vi "FTW-Regex.vi"(0 "Regular Expression":string, 5 "Input String":string, 9 "Starting Offset":i32, 11 "error in":errorcluster) -> (4 "Match":string, 6 "Submatches":string[](array[string]), 8 "Match Found?":bool, 10 "Offset after Match":i32, 15 "error out":errorcluster)   [LabVIEW 2013]
panel:
  out "Match Offsets":i32[](array[numeric])
  # "Inputs"
  # "Debug"
  # "Outputs"
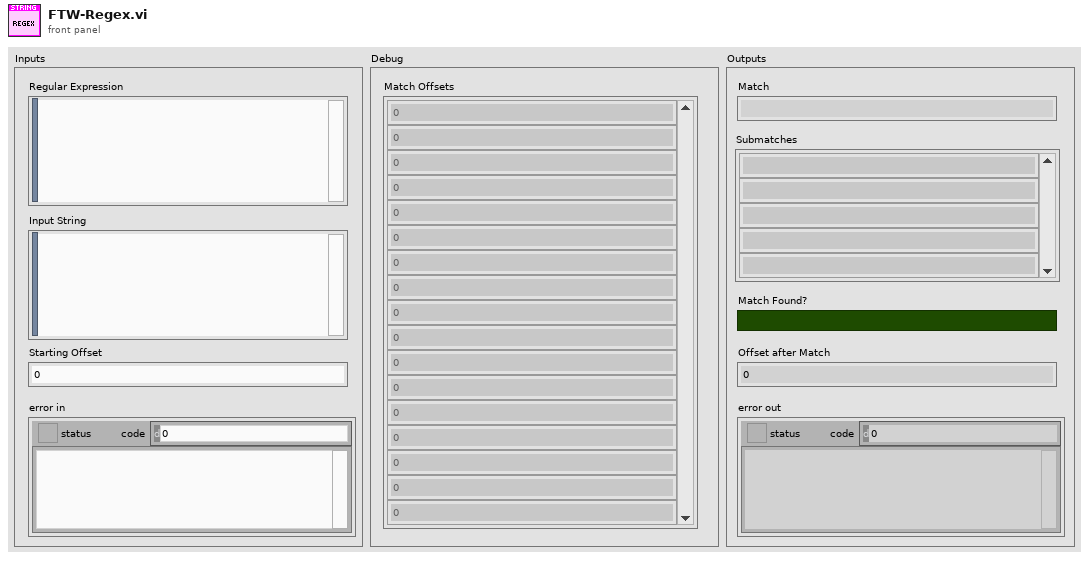
[diagram p1: front panel]
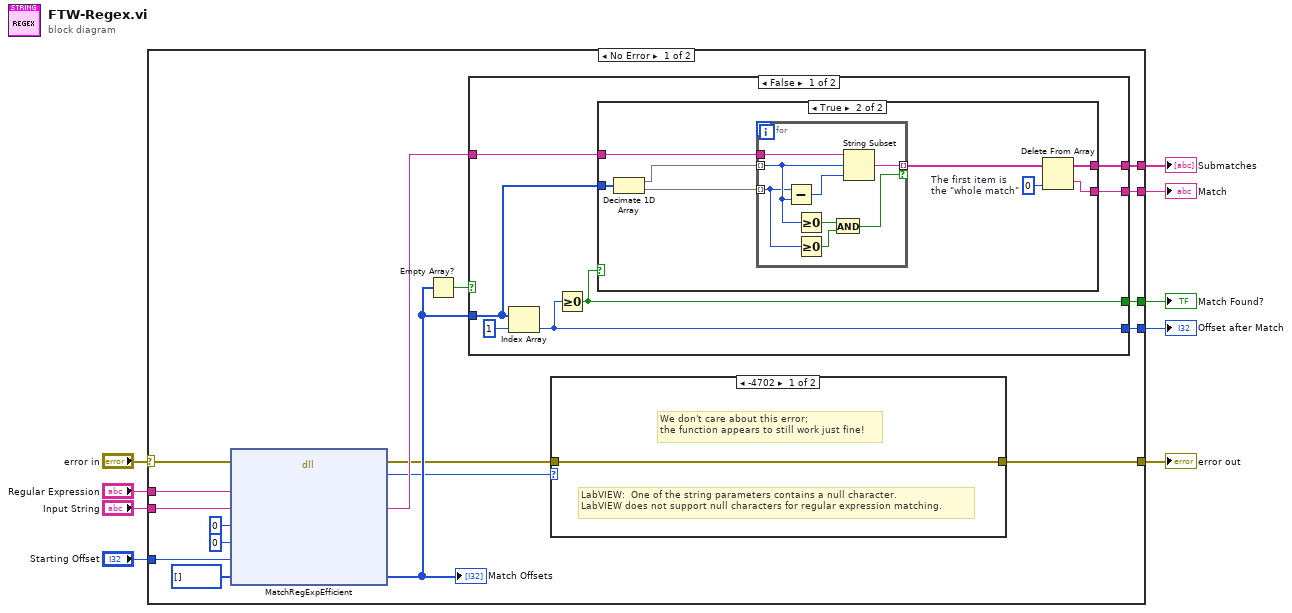
[diagram p0: block diagram]
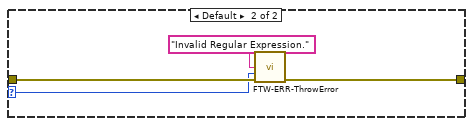
[diagram p2: hidden frame]
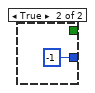
[diagram p4: hidden frame]
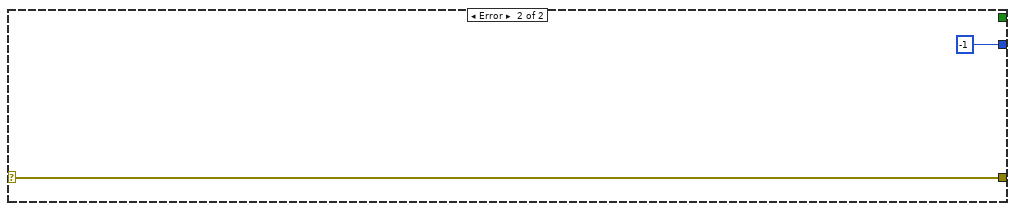
[diagram p5: hidden frame]
diagram:
  n1 = case shown="No Error" "error in" {
    selector: "error in" -> [w13 w56]
    tunnel: "Regular Expression" -> [w26 _]
    tunnel: [w25 _] -> w8
    tunnel: [w24 _] -> w7
    tunnel: [w11 w56] -> w6
    tunnel: "Starting Offset" -> [w23 _]
    tunnel: [w22 -1] -> w4
    tunnel: [w21 _] -> w3
    tunnel: "Input String" -> [w20 _]
    frame No Error {
      n2 = dll-call lib="LabVIEW" fn="MatchRegExpEfficient"(error in=w13, "Regular Expression"=w26, "Subject"=w20, "Ignore Case?"=0, "Multiline?"=0, "Starting Offset"=w23, "Match Offsets"=i32[] []) -> (error out=w12:errorcluster, "Return"=w10:i32, "Subject"=w19:string, "Match Offsets"=w15:i32[])  [unwired: 6 in, 1 out]
      "Match Offsets" <- w15
      n3 = Empty Array?(array=w15) -> (empty?=w14:bool)
      n4 = case shown="False" w14 {
        tunnel: [w38 _] -> w25
        tunnel: [w37 _] -> w24
        tunnel: [w35 -1] -> w22
        tunnel: [w34 _] -> w21
        tunnel: w19 -> [w33 _]
        tunnel: w15 -> [w32 _]
        frame False {
          n5 = Index Array(array=w32, index=1) -> (element=w35:i32)
          n6 = Greater Or Equal To 0?(x=w35) -> (x >= 0?=w34:bool)
          n7 = case shown="True" w34 {
            tunnel: w33 -> [_ w46]
            tunnel: [_ w42] -> w38
            tunnel: [_ w41] -> w37
            tunnel: w32 -> [_ w39]
            frame False {
            }
            frame True {
              w43 = 0  # The first item is the "whole match"
              n8 = Decimate 1D Array(w39) -> (w45:i32[], w40:i32[])
              n9 = for {
                tunnel: w46 -> [w54]
                tunnel: [w53] -> w44 mode=indexing if=w48
                tunnel: w45 -> [w51] mode=indexing
                tunnel: w40 -> [w47] mode=indexing
                n10 = Subtract(x=w47, y=w51) -> (x-y=w52:i32)
                n11 = Greater Or Equal To 0?(x=w51) -> (x >= 0?=w50:bool)
                n12 = Greater Or Equal To 0?(x=w47) -> (x >= 0?=w49:bool)
                n13 = And(x=w50, y=w49) -> (x .and. y?=w48:bool)
                n14 = String Subset(string=w54, offset (0)=w51, length (rest)=w52) -> (substring=w53:string)
              }
              n15 = Delete From Array(array=w44, index=w43) -> (deleted portion=w42:string, array with subset deleted=w41:string[])  [unwired: 1 in]
            }
          }
        }
        frame True {
        }
      }
      n16 = case shown="-4702" w10 {
        selector: w10 -> [_ w28]
        tunnel: w12 -> [w27 w31]
        tunnel: [w27 w30] -> w11
        frame -4702 {
          # "We don't care about this error;\nthe function appears to still work just fine!"
          # "LabVIEW:  One of the string parameters contains a null character.\nLabVIEW does not support null characters for regular expression matching."
        }
        frame Default {
          n17 = call "FTW-ERR-ThrowError.vi"("Error Message"="Invalid Regular Expression.", "Error Code"=w28, "error in"=w31) -> ("error out"=w30:errorcluster)  [unwired: 12 in]
        }
      }
    }
    frame Error {
    }
  }
  "error out" <- w6
  "Submatches" <- w7
  "Match" <- w8
  "Match Found?" <- w3
  "Offset after Match" <- w4
